vi "CAPTURE_STOP.vi"(2 "error in (no error)":errorcluster, 3 "VISA resource name":refnum<visa-resource-name>) -> (0 "error out":errorcluster, 1 "VISA resource Quit":refnum<visa-resource-name>)   [LabVIEW 2011]
panel:
  out "unsigned byte array":u8[](array[numeric])
  out "return count":u32
  out "Read command capture STOP":u8[](array[numeric])
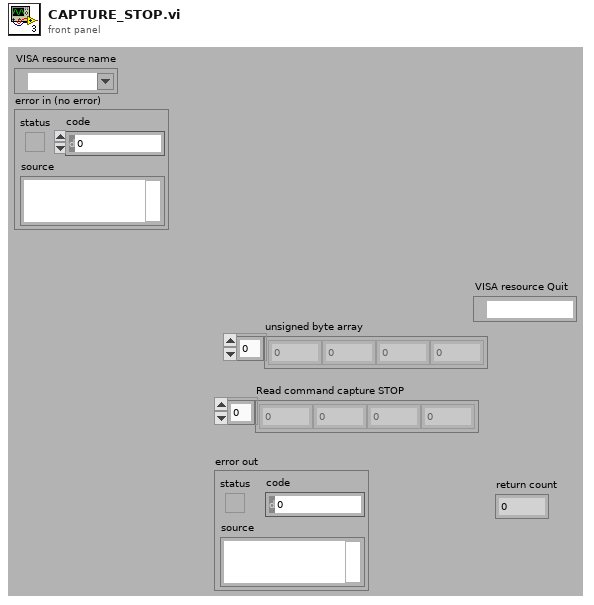
[diagram p1: front panel]
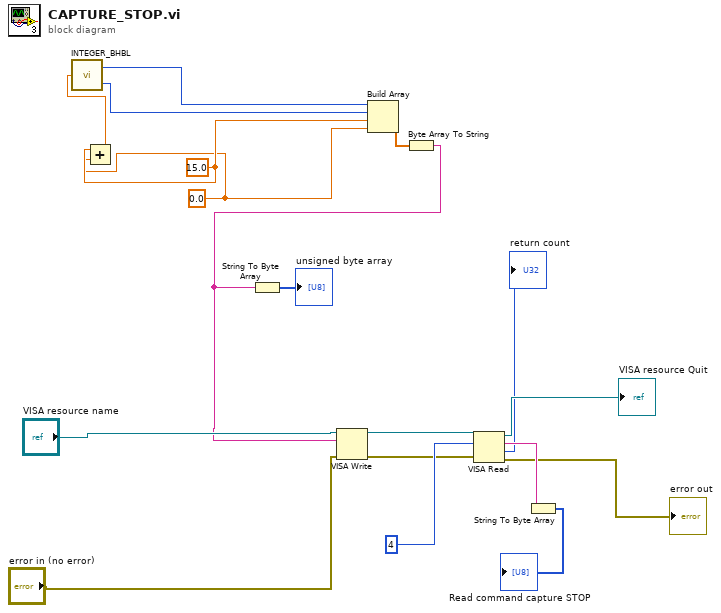
[diagram p0: block diagram]
diagram:
  w6 = 0.0 ("element")
  w7 = 15.0 ("element")
  n1 = Add(x=w7, y=w6) -> (x+y=w5:dbl)
  n2 = call "INTEGER_BHBL.vi"("int16"=w5) -> ("Lvalue"=w3:u8, "HValue"=w4:u8)
  n3 = Build Array(w4, w3, w7, w6) -> (w11:dbl[])
  n4 = Byte Array To String(unsigned byte array=w11) -> (string=w2:string)
  n5 = String To Byte Array(string=w2) -> (unsigned byte array=→"unsigned byte array":u8[])
  n6 = VISA Write(VISA resource name="VISA resource name", write buffer=w2, error in (no error)="error in (no error)") -> (VISA resource name out=w12:refnum<visa-resource-name>, error out=w14:errorcluster)  [unwired: 1 out]
  n7 = VISA Read(VISA resource name=w12, byte count=u32 4, error in (no error)=w14) -> (VISA resource name out=→"VISA resource Quit":refnum<visa-resource-name>, read buffer=w17:string, return count=→"return count":u32, error out=→"error out":errorcluster)
  n8 = String To Byte Array(string=w17) -> (unsigned byte array=→"Read command capture STOP":u8[])
